vi "Write_Master_Config.vi"(4 "error in (no error)":errorcluster, 6 "Present Configuration":T1, 7 "configuration file path":path) -> (0 "error out":errorcluster)   [LabVIEW 2015]
uses:
  <vilib>/Utility/config.llb/Write Key (String).vi
  <vilib>/Utility/config.llb/NI_LVConfig.lvlib
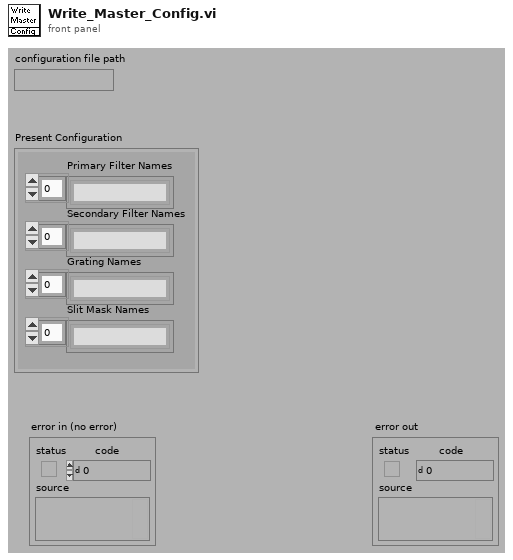
[diagram p1: front panel]
types:
  T1 = cluster{"Primary Filter Names":string[], "Secondary Filter Names":string[], "Grating Names":string[], "Slit Mask Names":string[]}
  T2 = typedef "NI_LVConfig.lvlib/Config Data RefNum.ctl" = refnum<k1>
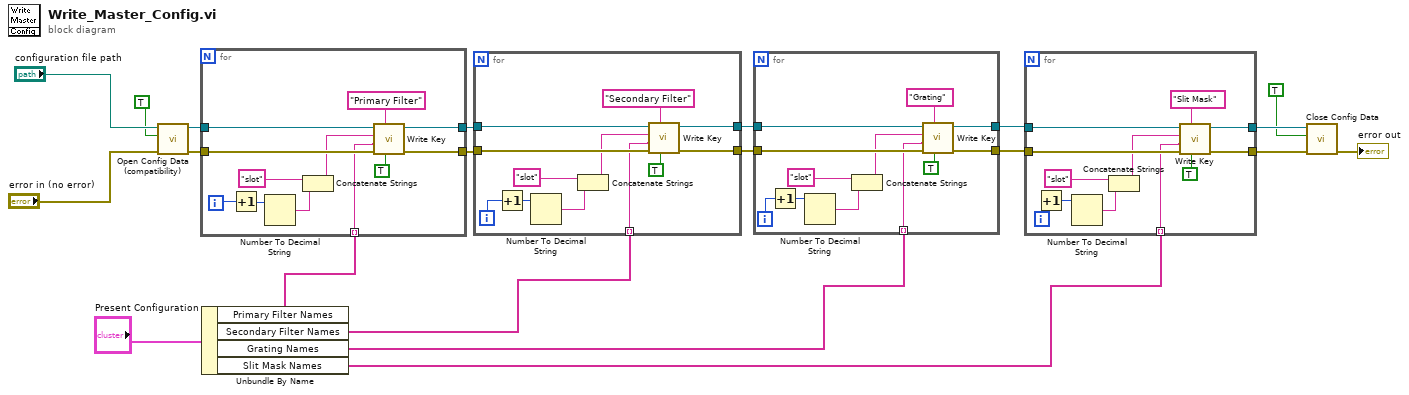
[diagram p0: block diagram]
diagram:
  n1 = call <vilib>:"Open Config Data (compatibility).vi"("error in (no error)"="error in (no error)", "create file if necessary (T)"=TRUE, "configuration file path"="configuration file path") -> ("error out"=w17:errorcluster, "refnum"=w16:T2)  [unwired: 6 in, 1 out]
  n2 = Unbundle By Name("Present Configuration") -> ("Primary Filter Names"=w4:string[], "Secondary Filter Names"=w3:string[], "Grating Names"=w2:string[], "Slit Mask Names"=w1:string[])
  n3 = for {
    tunnel: w17 -> [w32]
    tunnel: w16 -> [w31]
    tunnel: w4 -> [w26] mode=indexing
    tunnel: [w25] -> w15
    tunnel: [w24] -> w14
    i -> [w21]
    n4 = Increment(x=w21) -> (x+1=w22:i32)
    n5 = Number To Decimal String(number=w22) -> (decimal integer string=w29:string)  [unwired: 1 in]
    n6 = Concatenate Strings("slot", w29) -> (w27:string)
    n7 = call-poly <vilib>:"Write Key.vi"("write raw string? (F)"=TRUE, "section"="Primary Filter", "error in (no error)"=w32, "value"=w26, "key"=w27, "refnum"=w31) -> ("error out"=w25:errorcluster, "refnum out"=w24:T2)  [unwired: 3 in, 1 out]
  }
  n8 = for {
    tunnel: w15 -> [w44]
    tunnel: w14 -> [w43]
    tunnel: w3 -> [w38] mode=indexing
    tunnel: [w37] -> w13
    tunnel: [w36] -> w12
    i -> [w34]
    n9 = Increment(x=w34) -> (x+1=w33:i32)
    n10 = Number To Decimal String(number=w33) -> (decimal integer string=w41:string)  [unwired: 1 in]
    n11 = Concatenate Strings("slot", w41) -> (w39:string)
    n12 = call-poly <vilib>:"Write Key.vi"("write raw string? (F)"=TRUE, "section"="Secondary Filter", "error in (no error)"=w44, "value"=w38, "key"=w39, "refnum"=w43) -> ("error out"=w37:errorcluster, "refnum out"=w36:T2)  [unwired: 3 in, 1 out]
  }
  n13 = for {
    tunnel: w13 -> [w56]
    tunnel: w12 -> [w55]
    tunnel: w2 -> [w50] mode=indexing
    tunnel: [w49] -> w10
    tunnel: [w48] -> w11
    i -> [w45]
    n14 = Increment(x=w45) -> (x+1=w46:i32)
    n15 = Number To Decimal String(number=w46) -> (decimal integer string=w53:string)  [unwired: 1 in]
    n16 = Concatenate Strings("slot", w53) -> (w51:string)
    n17 = call-poly <vilib>:"Write Key.vi"("write raw string? (F)"=TRUE, "section"="Grating", "error in (no error)"=w56, "value"=w50, "key"=w51, "refnum"=w55) -> ("error out"=w49:errorcluster, "refnum out"=w48:T2)  [unwired: 3 in, 1 out]
  }
  n18 = for {
    tunnel: w10 -> [w68]
    tunnel: w11 -> [w67]
    tunnel: w1 -> [w62] mode=indexing
    tunnel: [w61] -> w8
    tunnel: [w60] -> w9
    i -> [w57]
    n19 = Increment(x=w57) -> (x+1=w58:i32)
    n20 = Number To Decimal String(number=w58) -> (decimal integer string=w65:string)  [unwired: 1 in]
    n21 = Concatenate Strings("slot", w65) -> (w63:string)
    n22 = call-poly <vilib>:"Write Key.vi"("write raw string? (F)"=TRUE, "section"="Slit Mask", "error in (no error)"=w68, "value"=w62, "key"=w63, "refnum"=w67) -> ("error out"=w61:errorcluster, "refnum out"=w60:T2)  [unwired: 3 in, 1 out]
  }
  n23 = call <vilib>:"Close Config Data.vi"("error in (no error)"=w8, "write file if changed (T)"=TRUE, "refnum"=w9) -> ("error out"=→"error out":errorcluster)  [unwired: 7 in, 1 out]
